vi "Run 2.vi"   [LabVIEW 2016]
uses:
  <vilib>/NXT/Block Support/NXT_ButtonSelector.ctl
  <vilib>/NXT/Dual Mode Library/Waits/Wait_Btn_Press.vi
types:
  T1 = typedef "NXT_ButtonSelector.ctl" = u16
  T2 = typedef "LVHSConnector.ctl" = refnum<class "BrickReference.lvclass">
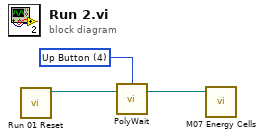
[diagram p0: block diagram]
diagram:
  w3 = T1 4 items=["Enter button"=3, "Left button"=2, "Right button"=1, "Up Button"=4, "Down Button"=5] ("Button (Enter button)")
  n1 = call "Run 01 Reset.vi"() -> ("NXT/EV3 out"=w2:T2)  [unwired: 11 in]
  n2 = call-poly <vilib>:"PolyWait.vi"("NXT/EV3"=w2, "Button (Enter button)"=w3) -> ("NXT/EV3"=w1:T2)  [unwired: 2 in]
  n3 = call "M07 Energy Cells.vi"("NXT/EV3"=w1) -> ()  [unwired: 11 in]
